vi "Run.vi"(10 "Return Queue":refnum<queue>, 11 "SessionHandler in":refnum<class "SessionHandler.lvclass">) -> ()   [LabVIEW 2017, in "Network Sink.lvlib" / "SessionHandler.lvclass"]
uses:
  <vilib>/gpm_packages/@cs/event-logger/Source/Network Sink/SessionHandler/SessionHandler.lvclass
  <vilib>/gpm_packages/@cs/event-logger/Source/Composed Log/Types/Log Level.ctl
  <vilib>/gpm_packages/@cs/event-logger/Source/Network Sink/SessionHandler/SessionHandler.lvclass/SessionHandler.ctl
  <vilib>/gpm_packages/@cs/event-logger/Source/Composed Log/Types/Log Packet.ctl
  <vilib>/gpm_packages/@cs/event-logger/Source/Composed Log/Composed Log.lvlib
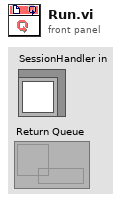
[diagram p1: front panel]
types:
  T1 = typedef "Composed Log.lvlib/Log Level.ctl" = enum16{"Debug", "Info", "Warning", "Error", "Critical"}
  T2 = typedef "Composed Log.lvlib/Log Packet.ctl" = cluster{"Data To Log":string, "Source":string, "Event Level":T1, "Event Time":timestamp}
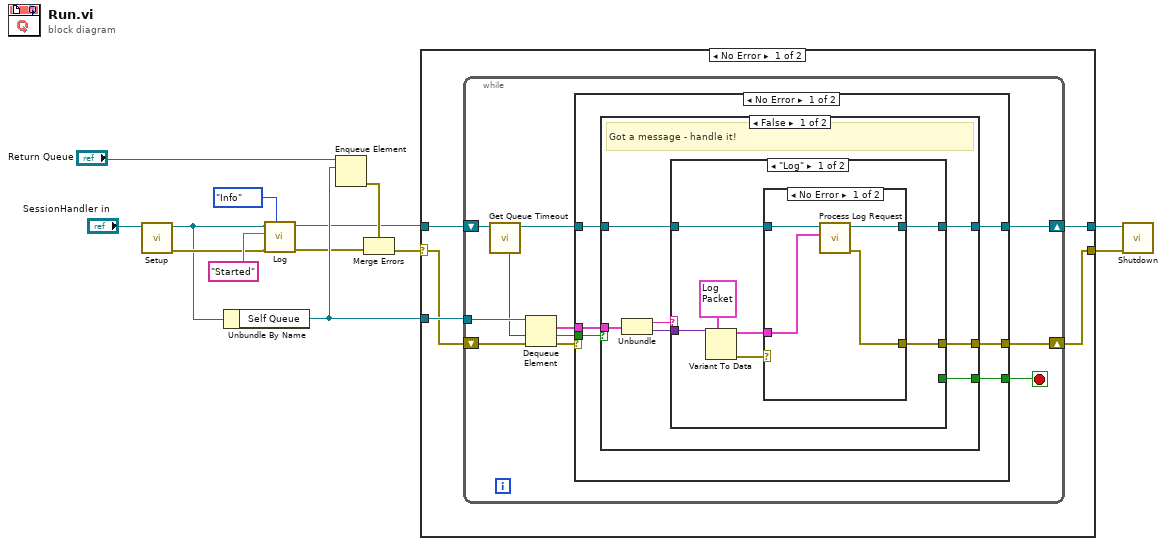
[diagram p0: block diagram]
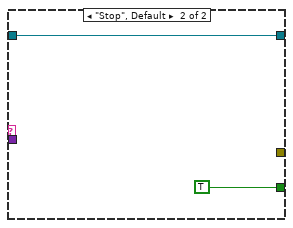
[diagram p3: hidden frame]
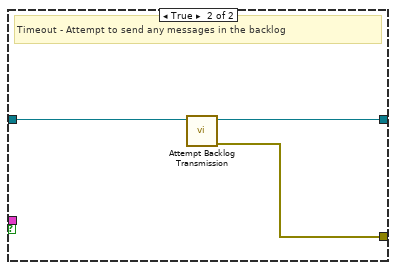
[diagram p4: hidden frame]
diagram:
  n1 = call <vilib>:"Setup.vi"("SessionHandler in"="SessionHandler in") -> ("error out"=w5:errorcluster, "SessionHandler out"=w4:refnum<class "SessionHandler.lvclass">)  [unwired: 9 in]
  n2 = Unbundle By Name(w4) -> ("Self Queue"=w11:refnum<queue>)
  n3 = call <vilib>:"Log.vi"("Event Level"=Log_Level."Info", "error in (no error)"=w5, "Data To Log"="Started", "SessionHandler in"=w4) -> ("error out"=w3:errorcluster, "SessionHandler out"=w2:refnum<class "SessionHandler.lvclass">)  [unwired: 6 in]
  n4 = Enqueue Element(queue="Return Queue", element=w11) -> (error out=w10:errorcluster)  [unwired: 2 in, 2 out]
  n5 = Merge Errors(w10, w3) -> (w9:errorcluster)
  n6 = case shown="No Error" w9 {
    selector: w9 -> [w14 w62]
    tunnel: w2 -> [w17 w63]
    tunnel: [w18 w63] -> w8
    tunnel: [w16 w62] -> w7
    tunnel: w11 -> [w15 _]
    frame No Error {
      n7 = while {
        shift-right: [w27] -> w18
        shift-left: w17 -> [w23]
        tunnel: w15 -> [w29]
        shift-right: [w24] -> w16
        shift-left: w14 -> [w19]
        stop <- w25 stop-if-true
        n8 = call <vilib>:"Get Queue Timeout.vi"("SessionHandler in"=w23) -> ("SessionHandler out"=w22:refnum<class "SessionHandler.lvclass">, "Queue Timeout"=w21:i32)  [unwired: 9 in]
        n9 = Dequeue Element(queue=w29, timeout in ms (-1)=w21, error in (no error)=w19) -> (element=w26:cluster{"Message":string, "Data":variant}, timed out?=w20:bool, error out=w28:errorcluster)  [unwired: 1 out]
        n10 = case shown="No Error" w28 {
          tunnel: w22 -> [w34 w61]
          tunnel: [w33 w61] -> w27
          tunnel: w26 -> [w35 _]
          tunnel: [w32 _] -> w25
          tunnel: [w31 _] -> w24
          tunnel: w20 -> [w30 _]
          frame No Error {
            n11 = case shown="False" w30 {
              tunnel: w35 -> [w42 _]
              tunnel: w34 -> [w41 w60]
              tunnel: [w40 w59] -> w33
              tunnel: [w37 _] -> w32
              tunnel: [w36 w58] -> w31
              frame False {
                # "Got a message - handle it!"
                n12 = Unbundle(w42) -> ("Message"=w39:string, "Data"=w38:variant)
                n13 = case shown="\"Log\"" w39 {
                  tunnel: w41 -> [w46 w57]
                  tunnel: [w45 w57] -> w40
                  tunnel: w38 -> [w49 _]
                  tunnel: [_ TRUE] -> w37
                  tunnel: [w43 _] -> w36
                  frame "Log" {
                    n14 = Variant To Data(type=T2 {"Data To Log"="", "Source"="", "Event Level"=enum."Debug", "Event Time"=timestamp(0 s since 1904-01-01)} ("Log Packet"), Variant=w49) -> (data=w44:T2, error out=w47:errorcluster)  [unwired: 1 in]
                    n15 = case shown="No Error" w47 {
                      selector: w47 -> [_ w54]
                      tunnel: w46 -> [w53 w55]
                      tunnel: [w52 w55] -> w45
                      tunnel: w44 -> [w51 _]
                      tunnel: [w50 w54] -> w43
                      frame No Error {
                        n16 = call-dynamic "Process Log Request.vi"("Log Packet"=w51, "SessionHandler in"=w53) -> ("error out"=w50:errorcluster, "SessionHandler out"=w52:refnum<class "SessionHandler.lvclass">)  [unwired: 8 in]
                      }
                      frame Error {
                      }
                    }
                  }
                  frame "Stop", Default {
                  }
                }
              }
              frame True {
                # "Timeout - Attempt to send any messages in the backlog"
                n17 = call <vilib>:"Attempt Backlog Transmission.vi"("SessionHandler in"=w60) -> ("error out"=w58:errorcluster, "SessionHandler out"=w59:refnum<class "SessionHandler.lvclass">)  [unwired: 9 in]
              }
            }
          }
          frame Error {
          }
        }
      }
    }
    frame Error {
    }
  }
  n18 = call <vilib>:"Shutdown.vi"("error in (no error)"=w7, "SessionHandler in"=w8) -> ()  [unwired: 10 in]
